vi "Import Routines.vi"(8 "error in (no error)":errorcluster, 11 "Node Ptr":u64 format="%.0x") -> (0 "error out":errorcluster)   [LabVIEW 2019, in "Diagnostics Addon System Explorer.lvlib"]
uses:
  Diagnostics Addon System Explorer.lvlib
  Types/Routine.Export.ctl
  Types/CmdResp.Export.ctl
  Shared/Types/Signal.ctl
  SubVIs/ID.FG.vi
  Shared/SubVIs/Constants.vi
  <vilib>/NI/NI VeriStand Advanced SysDef API/SysDef API/SysDef.CreateSection.vi
  <vilib>/NI/NI VeriStand Advanced SysDef API/SysDef API/SysDef.Property.Set.vi
  <vilib>/NI/NI VeriStand Advanced SysDef API/_SubVIs/SysDef.Property.Set.U32.vi
  <vilib>/NI VeriStand/Custom Device API/NI VeriStand - Get Item Property.vi
  <vilib>/NI VeriStand/Custom Device API/Get Item Property (U32).vi
  SubVIs/Service.Create.vi
  Shared/Diagnostics Addon Shared.lvlib
  <vilib>/NI VeriStand/Custom Device Tools/Custom Device Utility Library/Custom Device Utility Library.lvlib
  <vilib>/NI VeriStand/Custom Device API/Custom Device API.lvlib
panel:
  in  "Tag":string
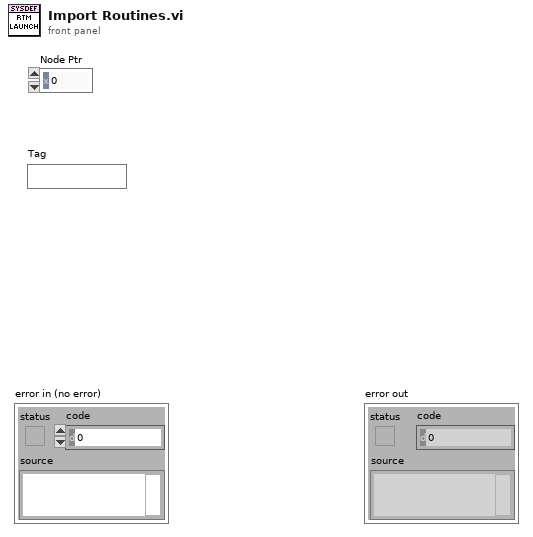
[diagram p1: front panel]
types:
  T1 = typedef "Diagnostics Addon System Explorer.lvlib/Routine.Export.ctl" = cluster{"Name":string, "ID":u16, "Start Parameters":T2, "Request Parameters":T2, "Stop Parameters":T2}
  T2 = typedef "Diagnostics Addon System Explorer.lvlib/CmdResp.Export.ctl" = cluster{"Cmd":T3[], "Response":T3[]}
  T3 = typedef "Diagnostics Addon Shared.lvlib/Signal.ctl" = cluster{"Start Bit":u32, "Length":u32, "Scaling Factor":dbl, "Scaling Offset":dbl, "Minimum":dbl, "Maximum":dbl, "Data Type":u32, "Byte Order":u32, "Default Value":dbl, "Name":string, "Units":string}
  T4 = typedef "Custom Device API.lvlib/Custom Device Item Ref.ctl" = u64
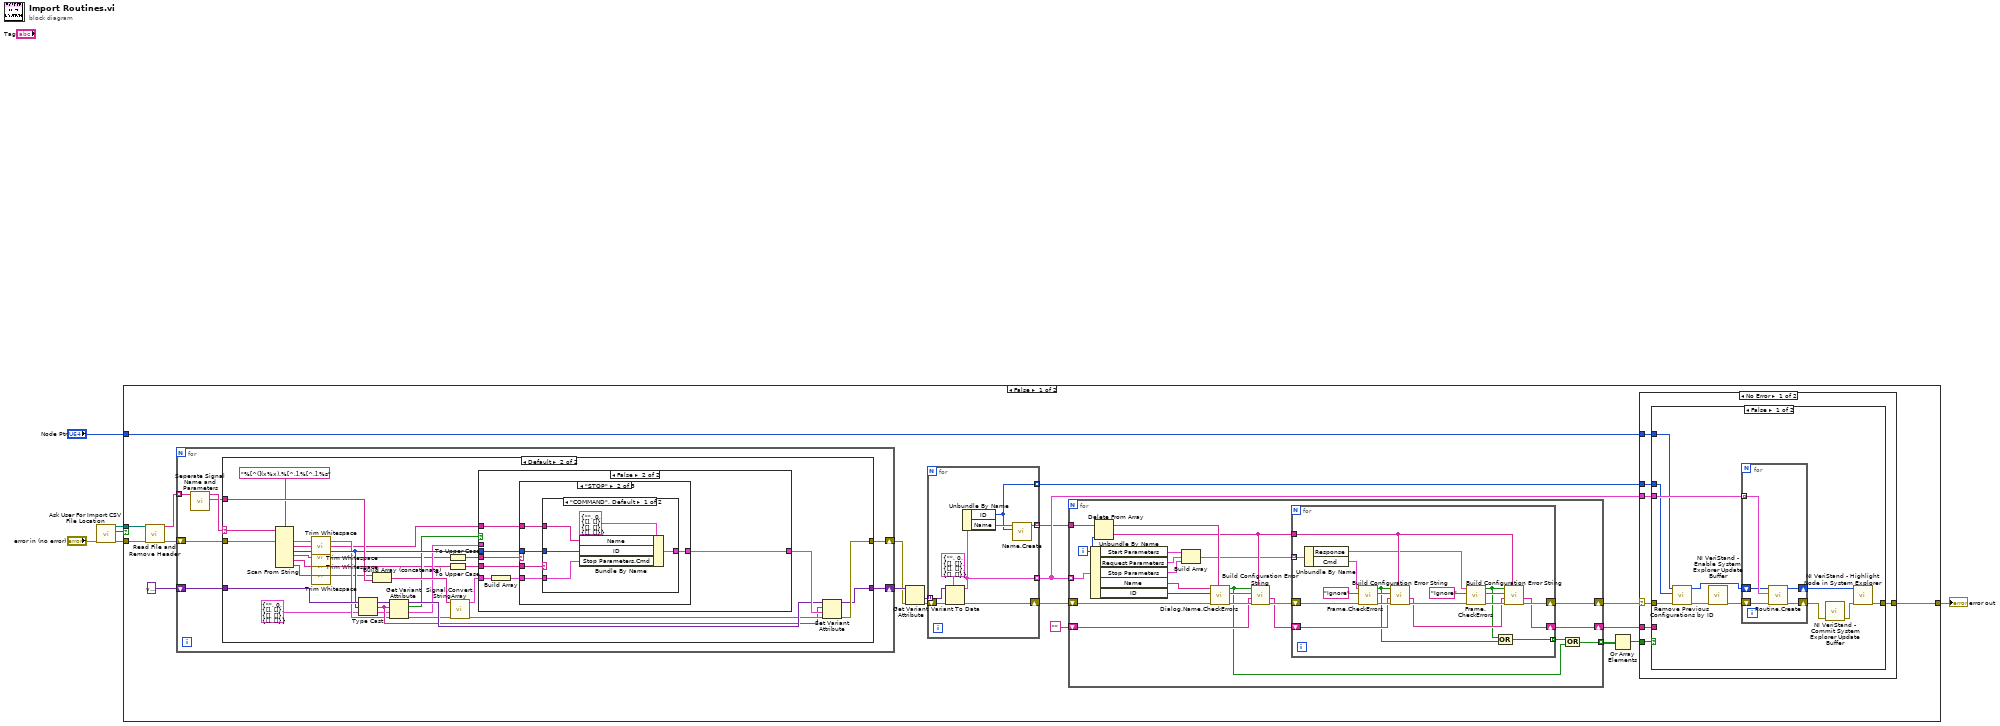
[diagram p0: block diagram]
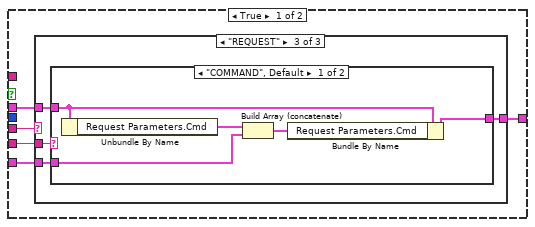
[diagram p3: hidden frame]
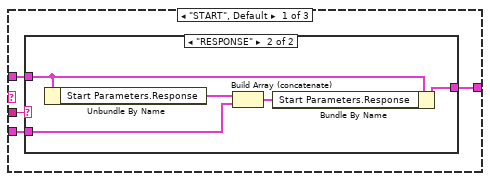
[diagram p4: hidden frame]
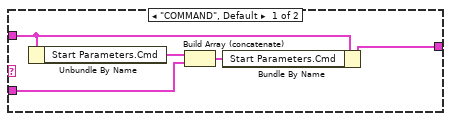
[diagram p5: hidden frame]
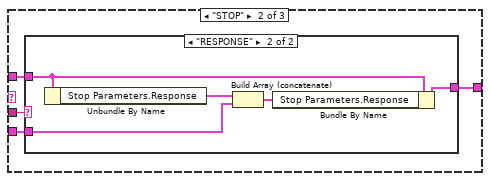
[diagram p6: hidden frame]
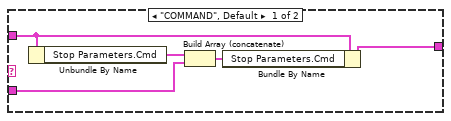
[diagram p7: hidden frame]
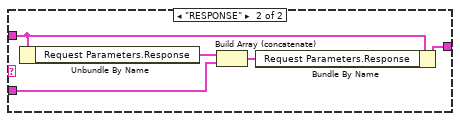
[diagram p8: hidden frame]
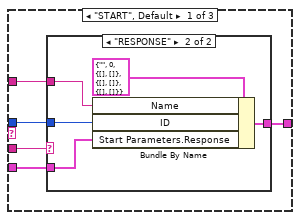
[diagram p9: hidden frame]
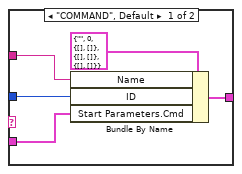
[diagram p10: hidden frame]
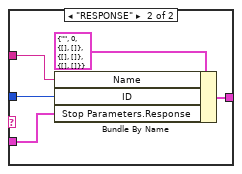
[diagram p11: hidden frame]
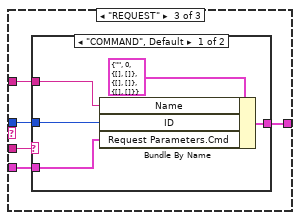
[diagram p12: hidden frame]
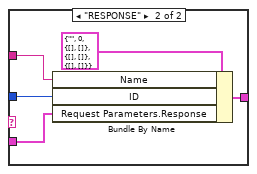
[diagram p13: hidden frame]
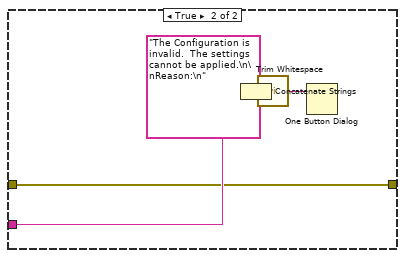
[diagram p14: hidden frame]
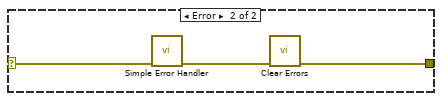
[diagram p15: hidden frame]
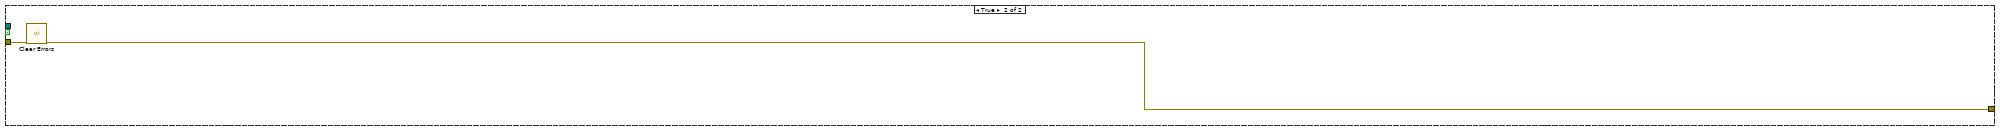
[diagram p16: hidden frame]
diagram:
  n1 = call "Ask User For Import CSV File Location.vi"("error in (no error)"="error in (no error)") -> ("error out"=w2:errorcluster, "cancelled"=w3:bool, "selected path"=w1:path)  [unwired: 8 in]
  n2 = case shown="False" w3 {
    tunnel: w2 -> [w26 w245]
    tunnel: w1 -> [w25 _]
    tunnel: "Node Ptr" -> [w11 _]
    tunnel: [w13 w244] -> w5
    frame False {
      n3 = call "Read File and Remove Header.vi"("error in (no error)"=w26, "selected path"=w25) -> ("error out"=w24:errorcluster, "Array"=w8:string[])  [unwired: 8 in]
      n4 = for {
        tunnel: w8 -> [w33] mode=indexing
        shift-right: [w30] -> w21
        shift-left: w24 -> [w31]
        shift-right: [w29] -> w22
        shift-left: variant -> [w32]
        n5 = call "Seperate Signal Name and Parameters.vi"("String"=w33) -> ("Signal Parameters"=w27:string[], "Signal Name"=w28:string)  [unwired: 9 in]
        n6 = case shown="Default" w28 {
          selector: w28 -> [_ w47]
          tunnel: w27 -> [_ w64]
          tunnel: w32 -> [w35 w60]
          tunnel: w31 -> [w34 w59]
          tunnel: [w34 w54] -> w30
          tunnel: [w35 w53] -> w29
          frame "" {
          }
          frame Default {
            n7 = Scan From String(format string="%[^(](x%x).%[^.].%[^.].%s", input string=w47, error in=w59) -> (error out=w51:errorcluster, output 1=w62:string, output 2=w58:u32, output 3=w45:string, output 4=w46:string, output 5=w41:string)  [unwired: 6 in, 2 out]
            n8 = call <vilib>:"Trim Whitespace.vi"("string"=w62) -> ("trimmed string"=w42:string)  [unwired: 1 in]
            n9 = call <vilib>:"Trim Whitespace.vi"("string"=w45) -> ("trimmed string"=w38:string)  [unwired: 1 in]
            n10 = call <vilib>:"Trim Whitespace.vi"("string"=w46) -> ("trimmed string"=w39:string)  [unwired: 1 in]
            n11 = call <vilib>:"Trim Whitespace.vi"("string"=w41) -> ("trimmed string"=w40:string)  [unwired: 1 in]
            n12 = Type Cast(x=w58) -> (*(type *) &x=w52:string)  [unwired: 1 in]
            n13 = Build Array (concatenate)(w40, w64) -> (w61:string[])
            n14 = Get Variant Attribute(Variant=w60, name=w52, default value (empty Variant)=T1 {"Name"="", "ID"=0, "Start Parameters"={"Cmd"=[], "Response"=[]}, "Request Parameters"={"Cmd"=[], "Response"=[]}, "Stop Parameters"={"Cmd"=[], "Response"=[]}} ("Routine"), error in=w51) -> (duplicate Variant=w56:variant, found=w49:bool, value=w48:T1, error out=w50:errorcluster)
            n15 = To Upper Case(1:w38) -> (0:w36:string)
            n16 = To Upper Case(1:w39) -> (0:w44:string)
            n17 = call "Signal.Convert.StringArray.vi"("error in (no error)"=w50, "Signal Parameters"=w61) -> ("error out"=w55:errorcluster, "Signal Parameters"=w63:T3)  [unwired: 8 in]
            n18 = case shown="False" w49 {
              tunnel: w63 -> [w68 w118]
              tunnel: w42 -> [_ w117]
              tunnel: w58 -> [_ w115]
              tunnel: [w67 w114] -> w57
              tunnel: w48 -> [w69 _]
              tunnel: w44 -> [w66 w113]
              tunnel: w36 -> [w65 w112]
              frame True {
                n19 = case shown="\"REQUEST\"" w65 {
                  tunnel: w69 -> [w73 w87 w101]
                  tunnel: w68 -> [w72 w86 w100]
                  tunnel: [w71 w85 w99] -> w67
                  tunnel: w66 -> [w70 w84 w98]
                  frame "START", Default {
                    n20 = case shown="\"RESPONSE\"" w70 {
                      tunnel: w73 -> [w78 w83]
                      tunnel: w72 -> [w76 w81]
                      tunnel: [w74 w79] -> w71
                      frame "COMMAND", Default {
                        n21 = Unbundle By Name(w78) -> ("Start Parameters.Cmd"=w77:T3[])
                        n22 = Build Array (concatenate)(w77, w76) -> (w75:T3[])
                        n23 = Bundle By Name(cluster=w78, "Start Parameters.Cmd"=w75) -> (w74:T1)
                      }
                      frame "RESPONSE" {
                        n24 = Unbundle By Name(w83) -> ("Start Parameters.Response"=w82:T3[])
                        n25 = Build Array (concatenate)(w82, w81) -> (w80:T3[])
                        n26 = Bundle By Name(cluster=w83, "Start Parameters.Response"=w80) -> (w79:T1)
                      }
                    }
                  }
                  frame "STOP" {
                    n27 = case shown="\"RESPONSE\"" w84 {
                      tunnel: w87 -> [w92 w97]
                      tunnel: w86 -> [w90 w95]
                      tunnel: [w88 w93] -> w85
                      frame "COMMAND", Default {
                        n28 = Unbundle By Name(w92) -> ("Stop Parameters.Cmd"=w91:T3[])
                        n29 = Build Array (concatenate)(w91, w90) -> (w89:T3[])
                        n30 = Bundle By Name(cluster=w92, "Stop Parameters.Cmd"=w89) -> (w88:T1)
                      }
                      frame "RESPONSE" {
                        n31 = Unbundle By Name(w97) -> ("Stop Parameters.Response"=w96:T3[])
                        n32 = Build Array (concatenate)(w96, w95) -> (w94:T3[])
                        n33 = Bundle By Name(cluster=w97, "Stop Parameters.Response"=w94) -> (w93:T1)
                      }
                    }
                  }
                  frame "REQUEST" {
                    n34 = case shown="\"COMMAND\", Default" w98 {
                      tunnel: w101 -> [w106 w111]
                      tunnel: w100 -> [w104 w109]
                      tunnel: [w102 w107] -> w99
                      frame "COMMAND", Default {
                        n35 = Unbundle By Name(w106) -> ("Request Parameters.Cmd"=w105:T3[])
                        n36 = Build Array (concatenate)(w105, w104) -> (w103:T3[])
                        n37 = Bundle By Name(cluster=w106, "Request Parameters.Cmd"=w103) -> (w102:T1)
                      }
                      frame "RESPONSE" {
                        n38 = Unbundle By Name(w111) -> ("Request Parameters.Response"=w110:T3[])
                        n39 = Build Array (concatenate)(w110, w109) -> (w108:T3[])
                        n40 = Bundle By Name(cluster=w111, "Request Parameters.Response"=w108) -> (w107:T1)
                      }
                    }
                  }
                }
              }
              frame False {
                n41 = Build Array(w118) -> (w116:T3[])
                n42 = case shown="\"STOP\"" w112 {
                  tunnel: w117 -> [w123 w138 w153]
                  tunnel: w116 -> [w122 w137 w152]
                  tunnel: w115 -> [w121 w136 w151]
                  tunnel: [w120 w135 w150] -> w114
                  tunnel: w113 -> [w119 w134 w149]
                  frame "START", Default {
                    n43 = case shown="\"RESPONSE\"" w119 {
                      tunnel: w123 -> [w128 w133]
                      tunnel: w122 -> [w127 w132]
                      tunnel: w121 -> [w126 w131]
                      tunnel: [w125 w130] -> w120
                      frame "COMMAND", Default {
                        n44 = Bundle By Name(cluster=T1 {"Name"="", "ID"=0, "Start Parameters"={"Cmd"=[], "Response"=[]}, "Request Parameters"={"Cmd"=[], "Response"=[]}, "Stop Parameters"={"Cmd"=[], "Response"=[]}} ("Routine"), "Name"=w128, "ID"=w126, "Start Parameters.Cmd"=w127) -> (w125:T1)
                      }
                      frame "RESPONSE" {
                        n45 = Bundle By Name(cluster=T1 {"Name"="", "ID"=0, "Start Parameters"={"Cmd"=[], "Response"=[]}, "Request Parameters"={"Cmd"=[], "Response"=[]}, "Stop Parameters"={"Cmd"=[], "Response"=[]}} ("Routine"), "Name"=w133, "ID"=w131, "Start Parameters.Response"=w132) -> (w130:T1)
                      }
                    }
                  }
                  frame "STOP" {
                    n46 = case shown="\"COMMAND\", Default" w134 {
                      tunnel: w138 -> [w143 w148]
                      tunnel: w137 -> [w142 w147]
                      tunnel: w136 -> [w141 w146]
                      tunnel: [w140 w145] -> w135
                      frame "COMMAND", Default {
                        n47 = Bundle By Name(cluster=T1 {"Name"="", "ID"=0, "Start Parameters"={"Cmd"=[], "Response"=[]}, "Request Parameters"={"Cmd"=[], "Response"=[]}, "Stop Parameters"={"Cmd"=[], "Response"=[]}} ("Routine"), "Name"=w143, "ID"=w141, "Stop Parameters.Cmd"=w142) -> (w140:T1)
                      }
                      frame "RESPONSE" {
                        n48 = Bundle By Name(cluster=T1 {"Name"="", "ID"=0, "Start Parameters"={"Cmd"=[], "Response"=[]}, "Request Parameters"={"Cmd"=[], "Response"=[]}, "Stop Parameters"={"Cmd"=[], "Response"=[]}} ("Routine"), "Name"=w148, "ID"=w146, "Stop Parameters.Response"=w147) -> (w145:T1)
                      }
                    }
                  }
                  frame "REQUEST" {
                    n49 = case shown="\"COMMAND\", Default" w149 {
                      tunnel: w153 -> [w158 w163]
                      tunnel: w152 -> [w157 w162]
                      tunnel: w151 -> [w156 w161]
                      tunnel: [w155 w160] -> w150
                      frame "COMMAND", Default {
                        n50 = Bundle By Name(cluster=T1 {"Name"="", "ID"=0, "Start Parameters"={"Cmd"=[], "Response"=[]}, "Request Parameters"={"Cmd"=[], "Response"=[]}, "Stop Parameters"={"Cmd"=[], "Response"=[]}} ("Routine"), "Name"=w158, "ID"=w156, "Request Parameters.Cmd"=w157) -> (w155:T1)
                      }
                      frame "RESPONSE" {
                        n51 = Bundle By Name(cluster=T1 {"Name"="", "ID"=0, "Start Parameters"={"Cmd"=[], "Response"=[]}, "Request Parameters"={"Cmd"=[], "Response"=[]}, "Stop Parameters"={"Cmd"=[], "Response"=[]}} ("Routine"), "Name"=w163, "ID"=w161, "Request Parameters.Response"=w162) -> (w160:T1)
                      }
                    }
                  }
                }
              }
            }
            n52 = Set Variant Attribute(Variant=w56, name=w52, value=w57, error in=w55) -> (Variant out=w53:variant, error out=w54:errorcluster)  [unwired: 1 out]
          }
        }
      }
      n53 = Get Variant Attribute(Variant=w22, error in=w21) -> (values=w20:variant[], error out=w19:errorcluster)  [unwired: 2 in, 2 out]
      n54 = for {
        tunnel: w20 -> [w171] mode=indexing
        shift-right: [w169] -> w12
        shift-left: w19 -> [w170]
        tunnel: [w168] -> w14 mode=indexing
        tunnel: [w165] -> w10 mode=indexing
        tunnel: [w166] -> w7 mode=indexing
        n55 = Variant To Data(error in=w170, type=T1 {"Name"="", "ID"=0, "Start Parameters"={"Cmd"=[], "Response"=[]}, "Request Parameters"={"Cmd"=[], "Response"=[]}, "Stop Parameters"={"Cmd"=[], "Response"=[]}} ("Routine"), Variant=w171) -> (data=w168:T1, error out=w169:errorcluster)
        n56 = Unbundle By Name(w168) -> ("ID"=w165:u16, "Name"=w167:string)
        n57 = call "Name.Create.vi"("PID Number"=w165, "PID Name"=w167) -> ("VS Name"=w166:string)  [unwired: 9 in]
      }
      n58 = for {
        tunnel: w14 -> [w193] mode=indexing
        shift-right: [w192] -> w9
        shift-left: w12 -> [w186]
        shift-right: [w180] -> w15
        shift-left: "" -> [w182]
        tunnel: [w179] -> w17 mode=indexing
        tunnel: w7 -> [w191]
        i -> [w190]
        n59 = Unbundle By Name(w193) -> ("Start Parameters"=w177:T2, "Request Parameters"=w176:T2, "Stop Parameters"=w175:T2, "Name"=w188:string, "ID"=w187:u16)
        n60 = Delete From Array(array=w191, index=w190) -> (deleted portion=w178:string, array with subset deleted=w189:string[])  [unwired: 1 in]
        n61 = Build Array(w177, w176, w175) -> (w174:T2[])
        n62 = call "Dialog.Name.CheckErrors.vi"("Existing Frames"=w189, "error in (no error)"=w186, "ID"=w187, "Name"=w188) -> ("error out"=w185:errorcluster, "Error"=w184:string, "Error?"=w173:bool)  [unwired: 5 in]
        n63 = call "Build Configuration Error String.vi"("Name"=w178, "error in (no error)"=w185, "String in"=w182, "Error"=w184, "Error?"=w173) -> ("error out"=w183:errorcluster, "String out"=w181:string)  [unwired: 5 in]
        n64 = for {
          tunnel: w178 -> [w200]
          shift-right: [w212] -> w192
          shift-left: w183 -> [w209]
          shift-right: [w202] -> w180
          shift-left: w181 -> [w204]
          tunnel: w174 -> [w199] mode=indexing
          tunnel: [w194] -> w172 mode=indexing
          n65 = Unbundle By Name(w199) -> ("Response"=w197:T3[], "Cmd"=w198:T3[])
          n66 = call "Frame.CheckErrors.vi"("error in (no error)"=w209, "Name"="Ignore", "Signals"=w198) -> ("error out"=w208:errorcluster, "Error Type"=w207:string, "Error?"=w195:bool)  [unwired: 6 in]
          n67 = call "Build Configuration Error String.vi"("Name"=w200, "error in (no error)"=w208, "String in"=w204, "Error"=w207, "Error?"=w195) -> ("error out"=w206:errorcluster, "String out"=w203:string)  [unwired: 5 in]
          n68 = call "Frame.CheckErrors.vi"("error in (no error)"=w206, "Name"="Ignore", "Signals"=w197) -> ("error out"=w211:errorcluster, "Error Type"=w205:string, "Error?"=w196:bool)  [unwired: 6 in]
          n69 = Compound Arithmetic op=OR(w196, w195) -> (w194:bool)
          n70 = call "Build Configuration Error String.vi"("Name"=w200, "error in (no error)"=w211, "String in"=w203, "Error"=w205, "Error?"=w196) -> ("error out"=w212:errorcluster, "String out"=w202:string)  [unwired: 5 in]
        }
        n71 = Compound Arithmetic op=OR(w172, w173) -> (w179:bool[])
      }
      n72 = Or Array Elements(Boolean array=w17) -> (logical OR=w16:bool)
      n73 = case shown="No Error" w9 {
        selector: w9 -> [w215 w243]
        tunnel: w16 -> [w219 _]
        tunnel: w15 -> [w218 _]
        tunnel: w14 -> [w217 _]
        tunnel: [w216 w241] -> w13
        tunnel: w11 -> [w214 _]
        tunnel: w10 -> [w213 _]
        frame No Error {
          n74 = case shown="False" w219 {
            tunnel: w218 -> [_ w238]
            tunnel: w215 -> [w223 w237]
            tunnel: w217 -> [w226 _]
            tunnel: [w225 w237] -> w216
            tunnel: w214 -> [w222 _]
            tunnel: w213 -> [w224 _]
            frame False {
              n75 = call "Remove Previous Configurations by ID.vi"("error in (no error)"=w223, "Imported IDs"=w224, "Node In"=w222) -> ("error out"=w221:errorcluster, "Node Out"=w220:T4)  [unwired: 7 in]
              n76 = call <vilib>:"NI VeriStand - Enable System Explorer Update Buffer.vi"("error in (no error)"=w221) -> ("error out"=w229:errorcluster)  [unwired: 10 in]
              n77 = for {
                shift-right: [w231] -> w228
                shift-left: w229 -> [w232]
                shift-right: [w233] -> w230
                shift-left: w220 -> [w234]
                tunnel: w226 -> [w235] mode=indexing
                n78 = call "Routine.Create.vi"("error in (no error)"=w232, "Routine"=w235, "Section Ptr"=w234) -> ("error out"=w231:errorcluster, "Parent Ref out"=w233:T4)  [unwired: 7 in]
              }
              n79 = call <vilib>:"NI VeriStand - Commit System Explorer Update Buffer.vi"("error in (no error)"=w228) -> ("error out"=w227:errorcluster)  [unwired: 10 in]
              n80 = call <vilib>:"NI VeriStand - Highlight Node in System Explorer.vi"("error in (no error)"=w227, "Item Ref in"=w230) -> ("error out"=w225:errorcluster)  [unwired: 8 in, 1 out]
            }
            frame True {
              n81 = Concatenate Strings("The Configuration is invalid.  The settings cannot be applied.\n\nReason:\n" ("message"), w238) -> (w240:string)
              n82 = call <vilib>:"Trim Whitespace.vi"("string"=w240) -> ("trimmed string"=w236:string)  [unwired: 1 in]
              n83 = One Button Dialog(message=w236) -> ()  [unwired: 1 in, 1 out]
            }
          }
        }
        frame Error {
          n84 = call <vilib>:"Simple Error Handler.vi"("error in (no error)"=w243) -> ("error out"=w242:errorcluster)  [unwired: 4 in, 4 out]
          n85 = call <vilib>:"Clear Errors.vi"("error in (no error)"=w242) -> ("error out"=w241:errorcluster)  [unwired: 5 in, 1 out]
        }
      }
    }
    frame True {
      n86 = call <vilib>:"Clear Errors.vi"("error in (no error)"=w245) -> ("error out"=w244:errorcluster)  [unwired: 5 in, 1 out]
    }
  }
  "error out" <- w5
